vi "Say Hi Msg Callback.vi"(7 "Owner":refnum<class>, 11 "Message":refnum<class "Message.lvclass">) -> (0 "error out":errorcluster)   [LabVIEW 2020]
uses:
  WebSocket Test UI Refs/WebSocket Test UI Refs.lvclass
  482d1ba6-16e1-4a0b-ae57-1cef22fe3f74.vi
  lv-msg-simple/Stream-Simple-Msg/Message/Message.lvclass
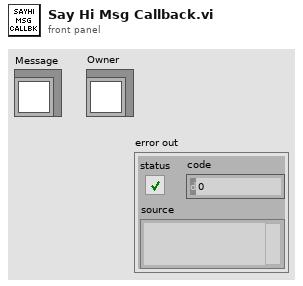
[diagram p1: front panel]
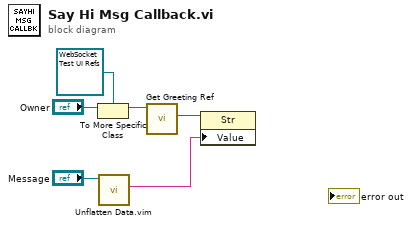
[diagram p0: block diagram]
diagram:
  n1 = To More Specific Class(target class=refnum<class "WebSocket Test UI Refs.lvclass"> refnum ("WebSocket Test UI Refs.lvclass"), reference="Owner") -> (specific class reference=w4:refnum<class "WebSocket Test UI Refs.lvclass">)  [unwired: 1 in, 1 out]
  n2 = call "Unflatten Data.vim"("Message in"="Message") -> ("Unflattened Data"=w1:string)  [unwired: 8 in, 2 out]
  n3 = call "Get Greeting Ref.vi"("WebSocket Test UI Refs in"=w4) -> ("Last Greeting"=w2:refnum<vi>)  [unwired: 8 in, 2 out]
  n4 = property class="Str"(reference=w2, "Value"=w1) -> ()  [unwired: 1 in, 2 out]
